vi "Accel Capture.vi"(10 "Capture Button Ref":refnum<vi>, 11 "Data IN":T1={"Message"="", "Homed?"=FALSE, "NextState"=enum."Timeout", "G.Load"=0.0, "G.Position"=0.0, "Load#"=0, "[G.Loads]"=[], "[TotalLoads]"=[], "[Errors]"=[], "ZeroWait"=0, "Results"=[], "DwellWait"=FALSE, "Test Result"=FALSE, "[CondyleLoads]"=[], "[Max]"=[], "[Min]"=[], "Valid String?"=FALSE, "ScanTime"=timestamp(0 s since 1904-01-01), "ScannedString"="", "LabelDevID"=0, "MfgDate"=timestamp(0 s since 1904-01-01), "[EEPROM Cmds]"=[], "[CalData]"=[], "[A/Ds]"=[], "[A/Dmax]"=[], "[A/Dmin]"=[], "BattMax"=0.0, "BattMin"=0.0, "DwellTime"=2000, "PendingDeviceType"="", "Zero G.load"=0.0, "GAINC Value"="", "Programming Step"=enum."Load EEPROM", "Front Panel Program?"=FALSE, "Final Program?"=FALSE, "PCB Score"=100, "AssyScore"=100, "Pass/Fail #"="", "Result String"="", "Programming Mode"=enum."Initial Program", "Angle Test Step"=enum."Initialize", "Accel Values"=[], "Shutdown Counter"=0, "V1"=0, "V2"=0, "V3"=0, "V4"=0, "EEPROM Data"=[], "Counter"=0, "Page#"=0, "Timer"=timestamp(0 s since 1904-01-01), "Use Mark10?"=FALSE, "Eng-Result#"=0, "DUT Serial #"=0, "Scroll Message?"=FALSE, "Clear Message"=FALSE, "Batt Test Step "=enum."Initialize", "RXTX Window Found?"=FALSE, "Shutdown First Call?"=FALSE, "A2 Delay (msec)"=500, "Support Script"={"Script #"="", "Script Revision"="", "[OEMs]"=[], "[[DeviceTypes]]"=[], "[[DeviceTypesVals]]"=[], "[[List of Errors]]"=[], "Default GAINC"="", "[[ASICtrims]]"=[], "ID For Echo"="", "Condyle A CalFactor"=100, "Condyle B CalFactor"=100, "[OEMs Prefix]"=[], "Packet ID 18"="", "[[Force Table Load Test]]"=[], "[[Force Table AccurTest]]"=[]}, "Serial Table"={"Serial File Path"=path "", "[[Serial Lookup Table]]"=[], "Serial Device Info"=[], "Valid Serial?"=FALSE}, "Target Information"={"Target Brand"="", "Target DeviceType"="", "Target Serial#"=100, "Target Lot#"=0, "Target DevID"=0, "Target Channel"=5}, "Operator"="", "COM Port"="", "Config Path"=path "", "Tx Array"=[], "DUT Parameters"={"Channel"=0, "DeviceID"=0, "Script Rev"=0, "Month"=0, "Day"=0, "Year"=0, "Lot#"=0, "V1"=0, "V2"=0, "V3"=0, "V4"=0, "MFG"=0, "Cal FactorA 10"=0, "Cal FactorB 10  "=0, "Cal FactorA 16"=0, "Cal FactorB 16"=0, "ASICtrim"=[], "TmpChan"=0, "GAINC"="", "Brand"="", "Device"="", "Serial #"=0, "Batt310"=0, "Batt 280"=0}, "FTS Main?"=FALSE, "Loading"={"[Forces]"=[], "[Dwell]"=[], "Loading Step"=enum."Initialize Test"}, "Software Version"="", "Correction Factor"="", "Second Load Test"=FALSE, "Acc Loads"=[], "Mark10 Config"={"H2S%"=[80.0, 85.0, 90.0, 95.0, 100.0], "H2S Speed"=[12.0, 8.0, 6.0, 4.0, 2.0], "H to S"=2.0, "Home Speed"=1.0, "LoadWin"=0.0, "Load Speed"=0.0, "PID"={"Kp"=0.04, "Kd"=0.005001, "Ki"=2.9999999999999923e-05}}, "Channels"={"Transceiver Ch"=5, "Operating Ch"=5, "Start Ch"=0}, "Channel EEPROM"=[], "Load Notes"=[], "Engr Log?"=FALSE, "Time"=[], "Program Retry"=FALSE, "Operator Channel"="", "Target Channel "="", "New Data Program"=FALSE, "NFHU Pass?"=FALSE, "Cycle Number"=0, "Cal Cycle#"=0, "[Avg G.Loads] "=[], "[Avg A/Ds] "=[], "Cal Retry?"=FALSE, "[Total A/Ds]  "=[], "Cycle Num LA"=0, "LA Cycle# "=0, "Shim Num"=0, "Shim#  "=0, "Angle Test?"=FALSE} {"Mark10 Config"."PID"."Ki" min=0.0 max=200.0 format="%.6f"; "Mark10 Config"."PID"."Kd" min=0.0 max=200.0 format="%.6f"; "Mark10 Config"."PID"."Kp" min=0.0 max=200.0 format="%.6f"; "DUT Parameters"."ASICtrim" format="%02x"}) -> (3 "Data Out":T1={"Message"="", "Homed?"=FALSE, "NextState"=enum."Timeout", "G.Load"=0.0, "G.Position"=0.0, "Load#"=0, "[G.Loads]"=[], "[TotalLoads]"=[], "[Errors]"=[], "ZeroWait"=0, "Results"=[], "DwellWait"=FALSE, "Test Result"=FALSE, "[CondyleLoads]"=[], "[Max]"=[], "[Min]"=[], "Valid String?"=FALSE, "ScanTime"=timestamp(0 s since 1904-01-01), "ScannedString"="", "LabelDevID"=0, "MfgDate"=timestamp(0 s since 1904-01-01), "[EEPROM Cmds]"=[], "[CalData]"=[], "[A/Ds]"=[], "[A/Dmax]"=[], "[A/Dmin]"=[], "BattMax"=0.0, "BattMin"=0.0, "DwellTime"=2000, "PendingDeviceType"="", "Zero G.load"=0.0, "GAINC Value"="", "Programming Step"=enum."Load EEPROM", "Front Panel Program?"=FALSE, "Final Program?"=FALSE, "PCB Score"=100, "AssyScore"=100, "Pass/Fail #"="", "Result String"="", "Programming Mode"=enum."Initial Program", "Angle Test Step"=enum."Initialize", "Accel Values"=[], "Shutdown Counter"=0, "V1"=0, "V2"=0, "V3"=0, "V4"=0, "EEPROM Data"=[], "Counter"=0, "Page#"=0, "Timer"=timestamp(0 s since 1904-01-01), "Use Mark10?"=FALSE, "Eng-Result#"=0, "DUT Serial #"=0, "Scroll Message?"=FALSE, "Clear Message"=FALSE, "Batt Test Step "=enum."Initialize", "RXTX Window Found?"=FALSE, "Shutdown First Call?"=FALSE, "A2 Delay (msec)"=500, "Support Script"={"Script #"="", "Script Revision"="", "[OEMs]"=[], "[[DeviceTypes]]"=[], "[[DeviceTypesVals]]"=[], "[[List of Errors]]"=[], "Default GAINC"="", "[[ASICtrims]]"=[], "ID For Echo"="", "Condyle A CalFactor"=100, "Condyle B CalFactor"=100, "[OEMs Prefix]"=[], "Packet ID 18"="", "[[Force Table Load Test]]"=[], "[[Force Table AccurTest]]"=[]}, "Serial Table"={"Serial File Path"=path "", "[[Serial Lookup Table]]"=[], "Serial Device Info"=[], "Valid Serial?"=FALSE}, "Target Information"={"Target Brand"="", "Target DeviceType"="", "Target Serial#"=100, "Target Lot#"=0, "Target DevID"=0, "Target Channel"=5}, "Operator"="", "COM Port"="", "Config Path"=path "", "Tx Array"=[], "DUT Parameters"={"Channel"=0, "DeviceID"=0, "Script Rev"=0, "Month"=0, "Day"=0, "Year"=0, "Lot#"=0, "V1"=0, "V2"=0, "V3"=0, "V4"=0, "MFG"=0, "Cal FactorA 10"=0, "Cal FactorB 10  "=0, "Cal FactorA 16"=0, "Cal FactorB 16"=0, "ASICtrim"=[], "TmpChan"=0, "GAINC"="", "Brand"="", "Device"="", "Serial #"=0, "Batt310"=0, "Batt 280"=0}, "FTS Main?"=FALSE, "Loading"={"[Forces]"=[], "[Dwell]"=[], "Loading Step"=enum."Initialize Test"}, "Software Version"="", "Correction Factor"="", "Second Load Test"=FALSE, "Acc Loads"=[], "Mark10 Config"={"H2S%"=[80.0, 85.0, 90.0, 95.0, 100.0], "H2S Speed"=[12.0, 8.0, 6.0, 4.0, 2.0], "H to S"=2.0, "Home Speed"=1.0, "LoadWin"=0.0, "Load Speed"=0.0, "PID"={"Kp"=0.04, "Kd"=0.005001, "Ki"=2.9999999999999923e-05}}, "Channels"={"Transceiver Ch"=5, "Operating Ch"=5, "Start Ch"=0}, "Channel EEPROM"=[], "Load Notes"=[], "Engr Log?"=FALSE, "Time"=[], "Program Retry"=FALSE, "Operator Channel"="", "Target Channel "="", "New Data Program"=FALSE, "NFHU Pass?"=FALSE, "Cycle Number"=0, "Cal Cycle#"=0, "[Avg G.Loads] "=[], "[Avg A/Ds] "=[], "Cal Retry?"=FALSE, "[Total A/Ds]  "=[], "Cycle Num LA"=0, "LA Cycle# "=0, "Shim Num"=0, "Shim#  "=0, "Angle Test?"=FALSE} {"Mark10 Config"."PID"."Ki" min=0.0 max=200.0 format="%.6f"; "Mark10 Config"."PID"."Kd" min=0.0 max=200.0 format="%.6f"; "Mark10 Config"."PID"."Kp" min=0.0 max=200.0 format="%.6f"; "DUT Parameters"."ASICtrim" format="%02x"})   [LabVIEW 2015]
uses:
  Controls/LocalVars.ctl
  Controls/Gen2 FT states.ctl
  Controls/Iniial Device Programming.ctl
  ProgramStageControl.ctl
  Controls/Batt Cap Steps.ctl
  Controls/Support Script.ctl
  Controls/Serial Table.ctl
  Controls/Device Information.ctl
  Controls/InfoPacket.ctl
  Controls/Loading.ctl
  Controls/Load Step.ctl
  Controls/Mark10 Config.ctl
  Controls/PID parameters.ctl
  Controls/Channels.ctl
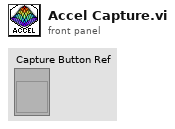
[diagram p1: front panel]
types:
  T1 = typedef "LocalVars.ctl" = cluster{"Message":string, "Homed?":bool, "NextState":T2, "G.Load":dbl, "G.Position":dbl, "Load#":i32, "[G.Loads]":dbl[], "[TotalLoads]":dbl[], "[Errors]":dbl[][], "ZeroWait":u32, "Results":dbl[], "DwellWait":bool, "Test Result":bool, "[CondyleLoads]":dbl[][], "[Max]":dbl[], "[Min]":dbl[], "Valid String?":bool, "ScanTime":timestamp, "ScannedString":string, "LabelDevID":u32, "MfgDate":timestamp, "[EEPROM Cmds]":u8[][], "[CalData]":u8[][], "[A/Ds]":dbl[][], "[A/Dmax]":dbl[], "[A/Dmin]":dbl[], "BattMax":dbl, "BattMin":dbl, "DwellTime":i32, "PendingDeviceType":string, "Zero G.load":dbl, "GAINC Value":string, "Programming Step":T3, "Front Panel Program?":bool, "Final Program?":bool, "PCB Score":i32, "AssyScore":i32, "Pass/Fail #":string, "Result String":string, "Programming Mode":T4, "Angle Test Step":enum16{"Initialize", "Get X", "Get Y", "Get Z", "Next Test"}, "Accel Values":dbl[][], "Shutdown Counter":u32, "V1":i32, "V2":i32, "V3":i32, "V4":i32, "EEPROM Data":i32[][], "Counter":i32, "Page#":i32, "Timer":timestamp, "Use Mark10?":bool, "Eng-Result#":u32, "DUT Serial #":i32, "Scroll Message?":bool, "Clear Message":bool, "Batt Test Step ":T5, "RXTX Window Found?":bool, "Shutdown First Call?":bool, "A2 Delay (msec)":i16, "Support Script":T6, "Serial Table":T7, "Target Information":T8, "Operator":string, "COM Port":string, "Config Path":path, "Tx Array":u8[], "DUT Parameters":T9, "FTS Main?":bool, "Loading":T10, "Software Version":string, "Correction Factor":string, "Second Load Test":bool, "Acc Loads":dbl[][], "Mark10 Config":T12, "Channels":T14, "Channel EEPROM":i32[][], "Load Notes":string[], "Engr Log?":bool, "Time":timestamp[], "Program Retry":bool, "Operator Channel":string, "Target Channel ":string, "New Data Program":bool, "NFHU Pass?":bool, "Cycle Number":i32, "Cal Cycle#":i32, "[Avg G.Loads] ":dbl[], "[Avg A/Ds] ":dbl[][], "Cal Retry?":bool, "[Total A/Ds]  ":dbl[][], "Cycle Num LA":i32, "LA Cycle# ":i32, "Shim Num":i32, "Shim#  ":i32, "Angle Test?":bool}
  T2 = typedef "Gen2 FT states.ctl" = enum16{"---------SETUP-------", "Initialization", "Read Support Data", "Initialize Mark-10", "Initialize Transceiver", "------UTILITIES------", "Change DUT Channel", "Find RxTx Window", "Reset Device", "Scan Channels", "Read Serial Lookup", "Shutdown Device", "ESTOP", "--------USER---------", "Timeout", "-----PROGRAM-----", "Program Device", "------MARK10--------", "Go Home", "MoveUp", "MoveDown", "Goto Load", "Goto Position", "Stop Motor", "---------TESTS--------", "Start Test", "Angle Test", "Load Test", "Load Accuracy Test", "Battery Test", "------RESULTS-------", "End Test", "Display Result", "--------EXIT--------", "Exit"}
  T3 = typedef "Iniial Device Programming.ctl" = enum16{"Load EEPROM", "Send First A1", "Send EEPROM", "Send A1", "Check EEPROM Echo", "Verify transmission", "Programming Successful", "Programming Failed"}
  T4 = typedef "ProgramStageControl.ctl" = enum16{"Initial Program", "GainC", "Scales"}
  T5 = typedef "Batt Cap Steps.ctl" = enum16{"Initialize", "Collect 2.8 Volts", "Collect 3.1 Volts", "Check Results"}
  T6 = typedef "Support Script.ctl" = cluster{"Script #":string, "Script Revision":string, "[OEMs]":string[], "[[DeviceTypes]]":string[][], "[[DeviceTypesVals]]":u16[][], "[[List of Errors]]":string[][], "Default GAINC":string, "[[ASICtrims]]":u8[][], "ID For Echo":string, "Condyle A CalFactor":i32, "Condyle B CalFactor":i32, "[OEMs Prefix]":string[], "Packet ID 18":string, "[[Force Table Load Test]]":dbl[][], "[[Force Table AccurTest]]":dbl[][]}
  T7 = typedef "Serial Table.ctl" = cluster{"Serial File Path":path, "[[Serial Lookup Table]]":string[][], "Serial Device Info":string[], "Valid Serial?":bool}
  T8 = typedef "Device Information.ctl" = cluster{"Target Brand":string, "Target DeviceType":string, "Target Serial#":i32, "Target Lot#":u32, "Target DevID":u32, "Target Channel":u8}
  T9 = typedef "InfoPacket.ctl" = cluster{"Channel":u8, "DeviceID":u32, "Script Rev":u8, "Month":u8, "Day":u8, "Year":u8, "Lot#":u32, "V1":u16, "V2":u16, "V3":u16, "V4":u16, "MFG":u8, "Cal FactorA 10":u8, "Cal FactorB 10  ":u8, "Cal FactorA 16":u8, "Cal FactorB 16":u8, "ASICtrim":u8[], "TmpChan":u8, "GAINC":string, "Brand":string, "Device":string, "Serial #":u64, "Batt310":u16, "Batt 280":u16}
  T10 = typedef "Loading.ctl" = cluster{"[Forces]":dbl[], "[Dwell]":dbl[], "Loading Step":T11}
  T11 = typedef "Load Step.ctl" = enum16{"Initialize Test", "Go Home", "Detect Dev Surface", "Wait to zero Device", "Zero Device", "Do Test", "Test Result"}
  T12 = typedef "Mark10 Config.ctl" = cluster{"H2S%":dbl[], "H2S Speed":dbl[], "H to S":dbl, "Home Speed":dbl, "LoadWin":dbl, "Load Speed":dbl, "PID":T13}
  T13 = typedef "PID parameters.ctl" = cluster{"Kp":dbl, "Kd":dbl, "Ki":dbl}
  T14 = typedef "Channels.ctl" = cluster{"Transceiver Ch":u8, "Operating Ch":u8, "Start Ch":u8}
  T15 = enum16{"Initialize", "Get X", "Get Y", "Get Z", "Next Test"}
  T16 = enum8{"Enabled", "Disabled", "Disabled and Grayed Out"}
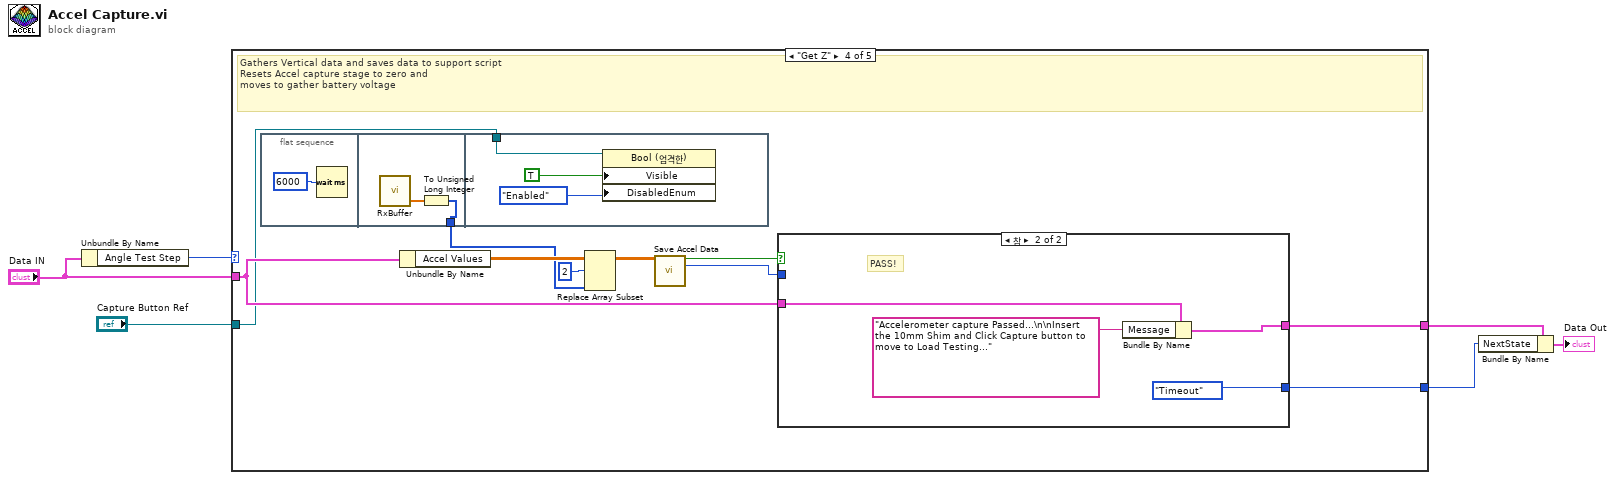
[diagram p0: block diagram]
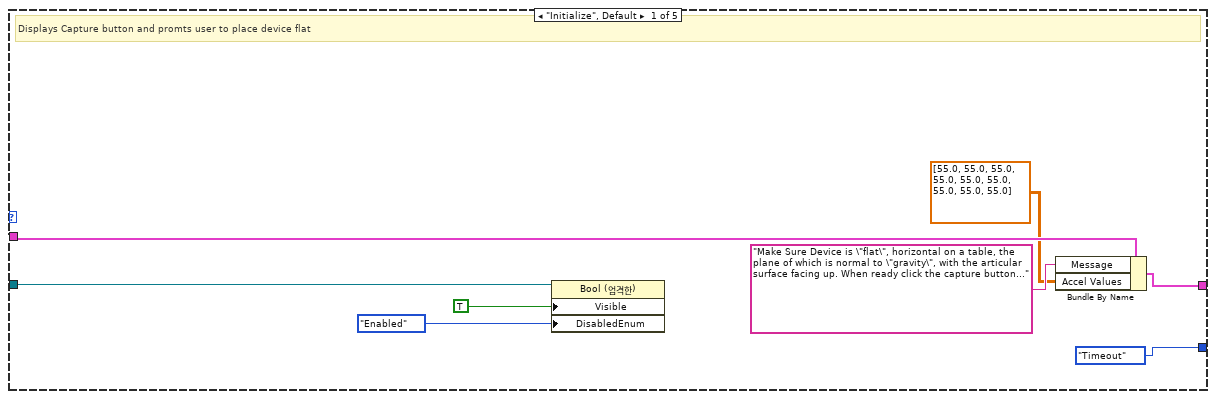
[diagram p2: hidden frame]
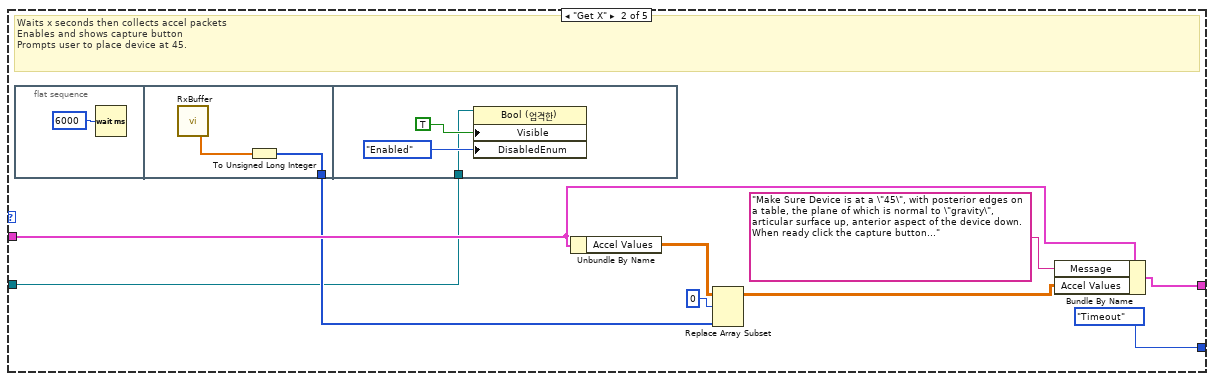
[diagram p3: hidden frame]
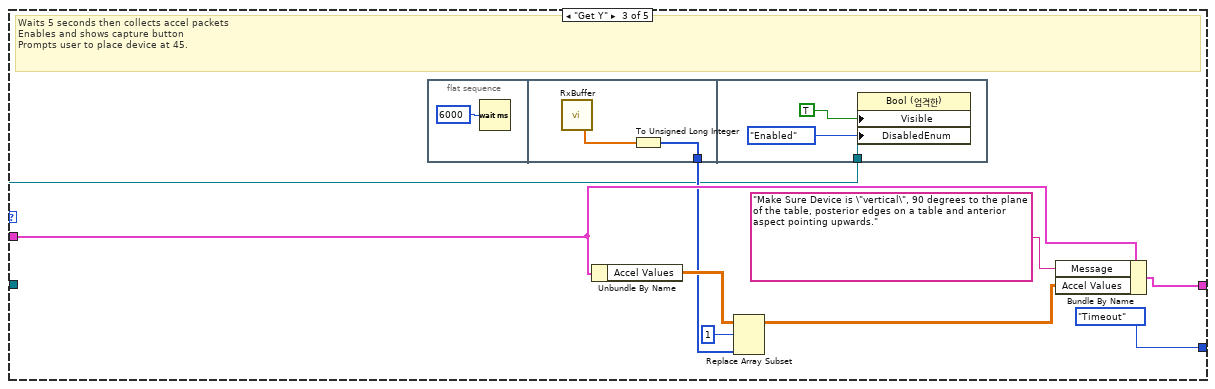
[diagram p4: hidden frame]
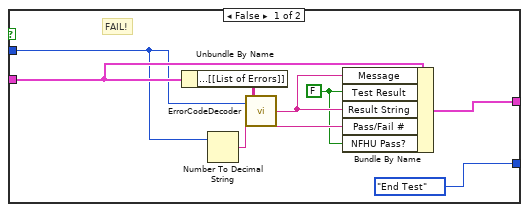
[diagram p5: hidden frame]
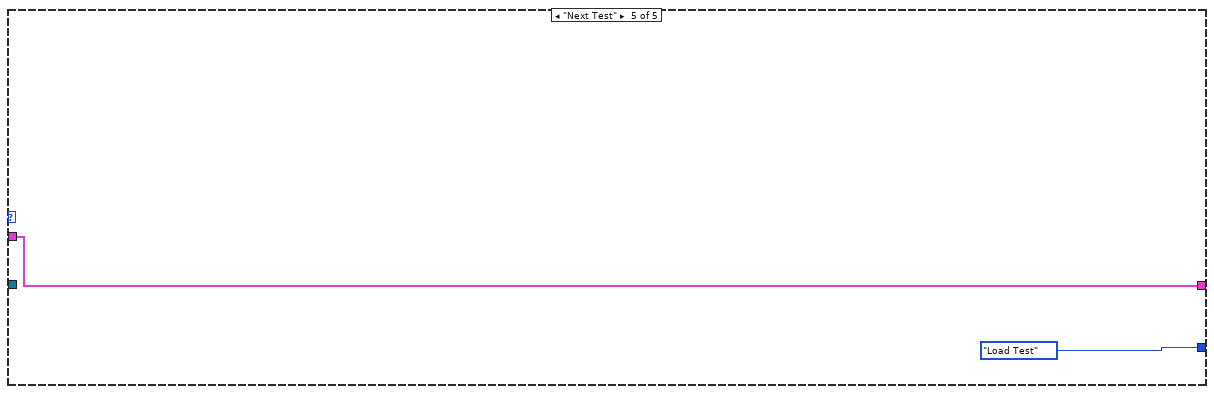
[diagram p6: hidden frame]
diagram:
  n1 = Unbundle By Name("Data IN") -> ("Angle Test Step"=w2:T15)
  n2 = case shown="\"Get Z\"" w2 {
    tunnel: [w10 w19 w35 w51 w73] -> w4
    tunnel: "Data IN" -> [w11 w20 w34 w47 w73]
    tunnel: [Gen2_FT_states."Timeout" ("NextState") Gen2_FT_states."Timeout" ("NextState") Gen2_FT_states."Timeout" ("NextState") w52 Gen2_FT_states."Load Test" ("NextState")] -> w6
    tunnel: "Capture Button Ref" -> [w7 w17 w30 w46 _]
    frame "Initialize", Default {
      # "Displays Capture button and promts user to place device flat"
      n3 = property on="Property Node" class="Bool (엄격한)"(reference=w7, "Visible"=TRUE, "DisabledEnum"=T16."Enabled" ("Disabled")) -> ()  [unwired: 1 in, 2 out]
      n4 = Bundle By Name(cluster=w11, "Message"="Make Sure Device is \"flat\", horizontal on a table, the plane of which is normal to \"gravity\", with the articular surface facing up. When ready click the capture button...", "Accel Values"=dbl[][] [[55.0, 55.0, 55.0], [55.0, 55.0, 55.0], [55.0, 55.0, 55.0]]) -> (w10:T1)
    }
    frame "Get X" {
      # "Waits x seconds then collects accel packets\nEnables and shows capture button\nPrompts user to place device at 45."
      n5 = flat-sequence {
        tunnel: [w25] -> w18
        tunnel: w17 -> [w27]
        frame #0 {
          n6 = Wait (ms)(milliseconds to wait=u32 6000) -> ()  [unwired: 1 out]
        }
        frame #1 {
          n7 = call "RxBuffer.vi"() -> ("Accelerometer"=w26:dbl[])  [unwired: 8 in, 11 out]
          n8 = To Unsigned Long Integer(number=w26) -> (unsigned 32bit integer=w25:u32[])
        }
        frame #2 {
          n9 = property on="Property Node" class="Bool (엄격한)"(reference=w27, "Visible"=TRUE, "DisabledEnum"=T16."Enabled" ("Disabled")) -> ()  [unwired: 1 in, 2 out]
        }
      }
      n10 = Unbundle By Name(w20) -> ("Accel Values"=w22:dbl[][])
      n11 = Replace Array Subset(array=w22, new element=w18, index (row)=0) -> (w16:dbl[][])  [unwired: 1 in]
      n12 = Bundle By Name(cluster=w20, "Message"="Make Sure Device is at a \"45\", with posterior edges on a table, the plane of which is normal to \"gravity\", articular surface up, anterior aspect of the device down. When ready click the capture button...", "Accel Values"=w16) -> (w19:T1)
    }
    frame "Get Y" {
      # "Waits 5 seconds then collects accel packets\nEnables and shows capture button\nPrompts user to place device at 45."
      n13 = flat-sequence {
        tunnel: [w40] -> w32
        tunnel: w30 -> [w42]
        frame #0 {
          n14 = Wait (ms)(milliseconds to wait=u32 6000) -> ()  [unwired: 1 out]
        }
        frame #1 {
          n15 = call "RxBuffer.vi"() -> ("Accelerometer"=w41:dbl[])  [unwired: 8 in, 11 out]
          n16 = To Unsigned Long Integer(number=w41) -> (unsigned 32bit integer=w40:u32[])
        }
        frame #2 {
          n17 = property on="Property Node" class="Bool (엄격한)"(reference=w42, "Visible"=TRUE, "DisabledEnum"=T16."Enabled" ("Disabled")) -> ()  [unwired: 1 in, 2 out]
        }
      }
      n18 = Unbundle By Name(w34) -> ("Accel Values"=w37:dbl[][])
      n19 = Replace Array Subset(array=w37, new element=w32, index (row)=1) -> (w31:dbl[][])  [unwired: 1 in]
      n20 = Bundle By Name(cluster=w34, "Message"="Make Sure Device is \"vertical\", 90 degrees to the plane of the table, posterior edges on a table and anterior aspect pointing upwards.", "Accel Values"=w31) -> (w35:T1)
    }
    frame "Get Z" {
      # "Gathers Vertical data and saves data to support script\nResets Accel capture stage to zero and\nmoves to gather battery voltage"
      n21 = flat-sequence {
        tunnel: [w68] -> w45
        tunnel: w46 -> [w72]
        frame #0 {
          n22 = Wait (ms)(milliseconds to wait=u32 6000) -> ()  [unwired: 1 out]
        }
        frame #1 {
          n23 = call "RxBuffer.vi"() -> ("Accelerometer"=w69:dbl[])  [unwired: 8 in, 11 out]
          n24 = To Unsigned Long Integer(number=w69) -> (unsigned 32bit integer=w68:u32[])
        }
        frame #2 {
          n25 = property on="Property Node" class="Bool (엄격한)"(reference=w72, "Visible"=TRUE, "DisabledEnum"=T16."Enabled" ("Disabled")) -> ()  [unwired: 1 in, 2 out]
        }
      }
      n26 = Unbundle By Name(w47) -> ("Accel Values"=w50:dbl[][])
      n27 = Replace Array Subset(array=w50, new element=w45, index (row)=2) -> (w48:dbl[][])  [unwired: 1 in]
      n28 = call "Save Accel Data.vi"("Accel Values"=w48) -> ("Pass?"=w53:bool, "Pass/Fail #"=w54:i32)  [unwired: 13 in]
      n29 = case shown="참" w53 {
        tunnel: [Gen2_FT_states."End Test" ("f") Gen2_FT_states."Timeout" ("f")] -> w52
        tunnel: [w60 w66] -> w51
        tunnel: w47 -> [w61 w64]
        tunnel: w54 -> [w57 _]
        frame False {
          w55 = FALSE ("Result")
          # "FAIL!"
          n30 = Unbundle By Name(w61) -> ("Support Script.[[List of Errors]]"=w62:string[][])
          n31 = Number To Decimal String(number=w57) -> (decimal integer string=w56:string)  [unwired: 1 in]
          n32 = call "ErrorCodeDecoder.vi"("array"=w62, "FTS Error Code In"=w57) -> ("Error Message"=w58:string)
          n33 = Bundle By Name(cluster=w61, "Message"=w58, "Test Result"=w55, "Result String"=w58, "Pass/Fail #"=w56, "NFHU Pass?"=w55) -> (w60:T1)
        }
        frame True {
          # "PASS!"
          n34 = Bundle By Name(cluster=w64, "Message"="Accelerometer capture Passed...\n\nInsert the 10mm Shim and Click Capture button to move to Load Testing...") -> (w66:T1)
        }
      }
    }
    frame "Next Test" {
    }
  }
  n35 = Bundle By Name(cluster=w4, "NextState"=w6) -> (→"Data Out":T1)
